vi "Initialize Motor.vi"(8 "error in (no error)":errorcluster, 10 "Axis:FMax":sgl=2.0, 11 "Device ID":T1) -> (0 "error out":errorcluster, 2 "Motor Error":i32, 3 "DC Motor Controller out":refnum<class "DC Motor Controller.lvclass">)   [LabVIEW 2012, in "UniCyRO.lvlib" / "UniCyRO_Host_Sim.lvclass"]
uses:
  UniCyRO_Host_Sim.lvclass
  <vilib>/robotics/Simulator/Engine/ctl/DeviceID.ctl
  <instrlib>/DC Motor Controller/HAIOL/DC Motor Controller.lvclass
  <vilib>/robotics/Simulator/Interface/Simulator References/Get Joint Reference (Hinge).vi
  <vilib>/robotics/Utilities/NI_Robotics Utilities.lvlib
  <instrlib>/DC Motor Controller/HAIOL/Simulator/DC Motor Controller Simulator.lvclass
  <vilib>/robotics/Simulator/NI_Robotics_Simulator.lvlib
  <resource>/objmgr/LVODE.rc
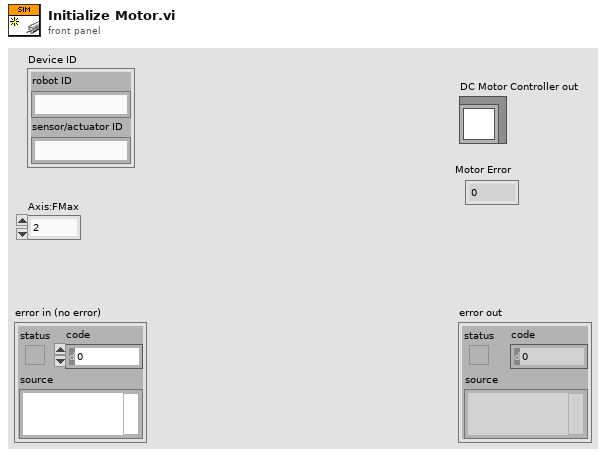
[diagram p1: front panel]
types:
  T1 = typedef "NI_Robotics_Simulator.lvlib/DeviceID.ctl" = cluster{"robot ID":string, "sensor/actuator ID":string}
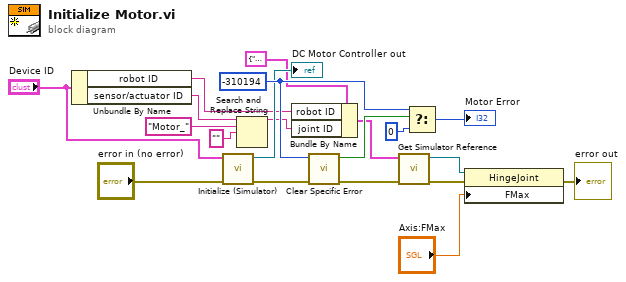
[diagram p0: block diagram]
diagram:
  w18 = -310194 ("code")
  n1 = Unbundle By Name("Device ID") -> ("robot ID"=w5:string, "sensor/actuator ID"=w4:string)
  n2 = call <instrlib>:"Initialize (Simulator).vi"("error in (no error)"="error in (no error)", "Device ID"="Device ID") -> ("error out"=w15:errorcluster, "DC Motor Controller out"=→"DC Motor Controller out":refnum<class "DC Motor Controller.lvclass">)  [unwired: 8 in]
  n3 = Search and Replace String(input string=w4, search string="Motor_", replace string="" ("replace string (\"\")")) -> (result string=w3:string)  [unwired: 5 in, 3 out]
  n4 = Bundle By Name(cluster=cluster{"robot ID":string, "joint ID":string} {"robot ID"="Sim Model 6_R0", "joint ID"="Motor_Drive Joint"} ("robot joint ID"), "robot ID"=w5, "joint ID"=w3) -> (w6:cluster{"robot ID":string, "joint ID":string})
  n5 = call <vilib>:"Clear Specific Error.vi"("error in (no error)"=w15, "code"=w18) -> ("error out"=w9:errorcluster, "code found?"=w19:bool)  [unwired: 7 in, 1 out]
  n6 = call-poly <vilib>:"Get Simulator Reference.vi"("error in (no error)"=w9, "robot joint ID"=w6) -> ("error out"=w12:errorcluster, "hinge joint ref"=w13:refnum<k20>)  [unwired: 8 in]
  n7 = Select(t=w18, s=w19, f=0) -> (s? t:f=→"Motor Error":i32)
  n8 = property class="HingeJoint"(reference=w13, error in=w12, "FMax"="Axis:FMax") -> (error out=→"error out":errorcluster)  [unwired: 1 out]
